vi "DSF.Engine.Pool.Set FIFO.vi"(10 "FIFO":refnum<k33>, 11 "Pool in":refnum<class "DSF.Engine.Pool.lvclass">) -> (3 "Pool out":refnum<class "DSF.Engine.Pool.lvclass">)   [LabVIEW 2016, in "DSF.Engine.lvlib" / "DSF.Engine.Pool.lvclass"]
uses:
  DSF.Engine.Pool.lvclass
  DSF.Engine.Pool.lvclass/DSF.Engine.Pool.ctl
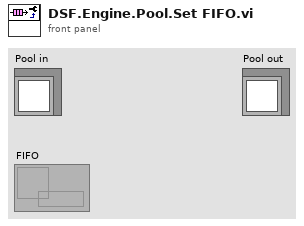
[diagram p1: front panel]
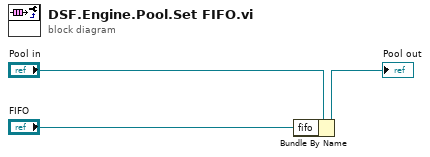
[diagram p0: block diagram]
diagram:
  n1 = Bundle By Name(cluster="Pool in", "fifo"="FIFO") -> (→"Pool out":refnum<class "DSF.Engine.Pool.lvclass">)
